vi "LEP_RV_GetSubTargetPath.vi"(1 "path":path) -> (0 "path":path)   [LabVIEW 2011]
uses:
  <vilib>/Platform/EmbProject/Plugins/utilities/LEP_Utilities_GetInfoGlobals.vi
  <vilib>/Platform/EmbProject/Plugins/utilities/LEP_Utilities_GetSetProjectData_String.vi
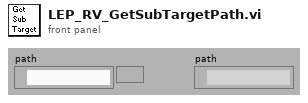
[diagram p1: front panel]
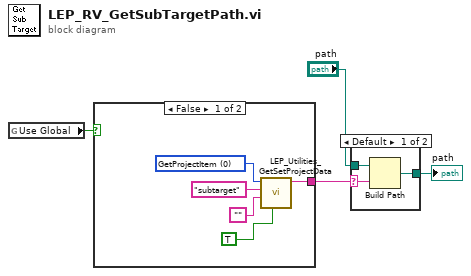
[diagram p0: block diagram]
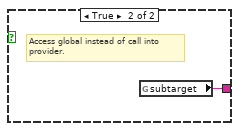
[diagram p2: hidden frame]
diagram:
  n1 = global read "LEP_Utilities_GetInfoGlobals.vi" "Use Global"() -> (w1:bool)
  n2 = case shown="False" w1 {
    tunnel: [w8 w10] -> w2
    frame False {
      w5 = u16 0 items=["GetProjectItem", "SetProjectItem"] ("Command")
      n3 = call-poly <vilib>:"LEP_Utilities_GetSetProjectData.vi"("access target data (F)"=TRUE, "data in"="", "ItemName"="subtarget", "Command"=w5) -> ("data out"=w8:string)  [unwired: 5 in, 2 out]
    }
    frame True {
      # "Access global instead of call into\nprovider."
      n4 = global read "LEP_Utilities_GetInfoGlobals.vi" "subtarget"() -> (w10:string)
    }
  }
  n5 = case shown="Default" w2 {
    selector: w2 -> [w12 _]
    tunnel: "path" -> [w13 w14]
    tunnel: [w11 w14] -> w4
    frame Default {
      n6 = Build Path(base path=w13, name or relative path=w12) -> (appended path=w11:path)
    }
    frame "" {
    }
  }
  "path" <- w4
